vi "Creators Status Created Queues.vi"(11 "Base Event jettl in":refnum<class "Base Event jettl.lvclass">) -> (0 "Created Queue Count":i32, 1 "Created Queue Aliases":string[](array[string]), 2 "Created Queue Exist?":bool, 3 "Base Event jettl out":refnum<class "Base Event jettl.lvclass">)   [LabVIEW 2021, in "jettl.lvlib" / "Base Event jettl.lvlib" / "Base Event jettl.lvclass"]
uses:
  Base Event jettl.lvclass
  C:/git/jettl/src/jettl/jettl/jettl.lvclass
  Base Event jettl.lvclass/Base Event jettl.ctl
  Queue Mailbox/Queue Mailbox.lvlib
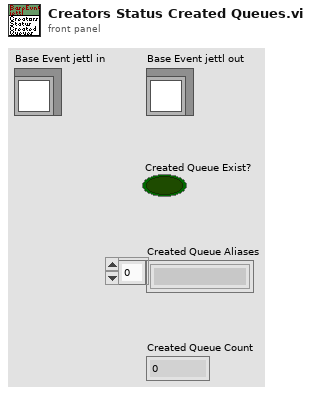
[diagram p1: front panel]
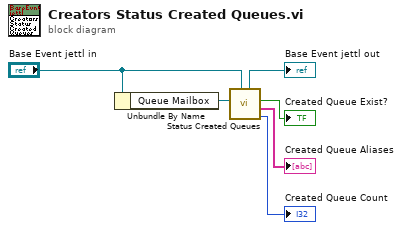
[diagram p0: block diagram]
diagram:
  n1 = Unbundle By Name("Base Event jettl in") -> ("Queue Mailbox"=w4:refnum<data-value>)
  n2 = call "Status Created Queues.vi"("jettl in"="Base Event jettl in", "Queue Mailbox"=w4) -> ("Created Queue Count"=→"Created Queue Count":i32, "Created Queue Aliases"=→"Created Queue Aliases":string[], "Created Queue Exist?"=→"Created Queue Exist?":bool, "jettl out"=→"Base Event jettl out":refnum<class "Base Event jettl.lvclass">)  [unwired: 6 in]
